vi "Eval_SglVar_MultiRes.vi"(8 "error in (no error)":errorcluster, 9 "varValue":dbl format="%#_13g", 11 "muExpr in":refnum<class "mupExpr.lvclass">) -> (0 "error out":errorcluster, 2 "Results":dbl[](array[numeric]), 3 "muExpr out":refnum<class "mupExpr.lvclass">)   [LabVIEW 2015, in "mupExpr.lvclass"]
doc: "Updates the value of the selected single variable then evaluates all expressions. Returns one result per expression.\n\nIf the expressions contain no variables, the input value is ignored.\n\nIf the expressions contain more than one variable only the \"Single Variable\" is updated.\n\nIf the variables are defined for bulk mode evaluation, only the first set (index 0) will be updated and evaluated."
uses:
  mupExpr.lvclass
  mupExpr.lvclass/mupExpr.ctl
  mupLib/mupCheckError.vi
  mupLib/mupLibPath.vi
  <vilib>/Utility/error.llb/Error Cluster From Error Code.vi
  mupLib/mupLib.lvlib
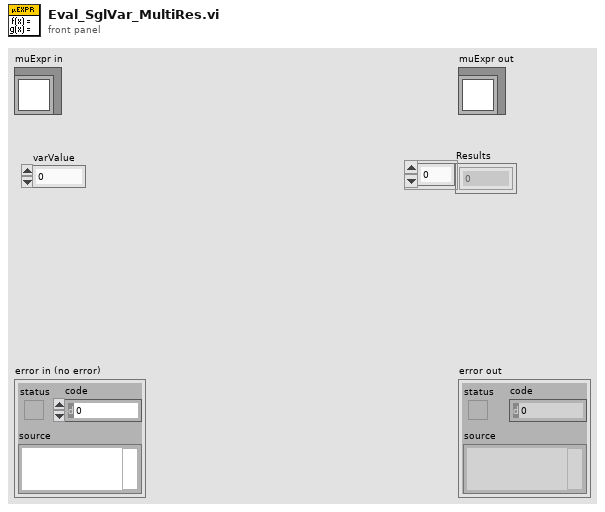
[diagram p1: front panel]
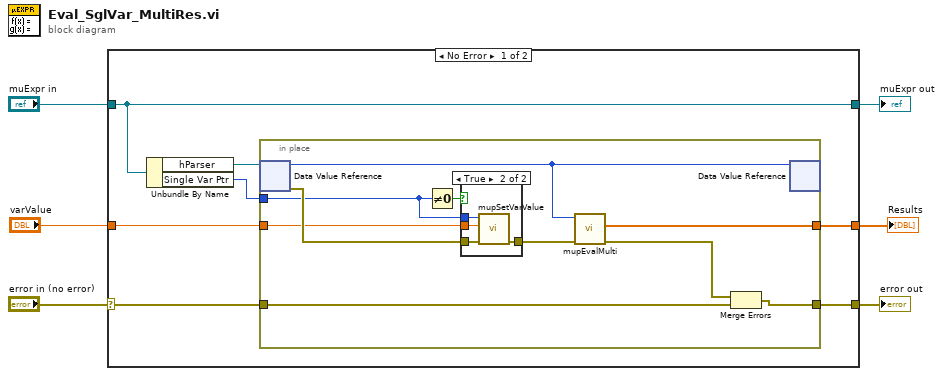
[diagram p0: block diagram]
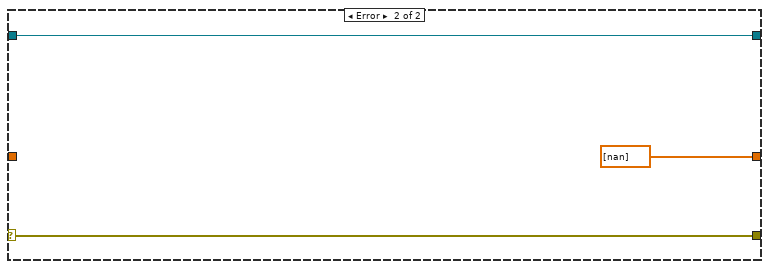
[diagram p3: hidden frame]
diagram:
  n1 = case shown="No Error" "error in (no error)" {
    selector: "error in (no error)" -> [w13 w31]
    tunnel: [w11 w31] -> w5
    tunnel: [w7 w30] -> w3
    tunnel: "muExpr in" -> [w7 w30]
    tunnel: "varValue" -> [w12 _]
    tunnel: [w10 dbl[] [nan] ("results")] -> w1
    frame No Error {
      n2 = Unbundle By Name(w7) -> ("hParser"=w9:refnum<data-value>, "Single Var Ptr"=w8:u64)
      n3 = in-place {
        in-place-border: w13 -> [w22]
        in-place-border: w12 -> [w16]
        in-place-border: [w20] -> w11
        in-place-border: [w23] -> w10
        in-place-border: w8 -> [w14]
        n4 = in-place-dvr #1(w9) -> (w15:u64, w17:errorcluster)
        n5 = Not Equal To 0?(x=w14) -> (x != 0?=w19:bool)
        n6 = case shown="True" w19 {
          tunnel: w17 -> [w24 w28]
          tunnel: w16 -> [_ w27]
          tunnel: [w24 w26] -> w18
          tunnel: w14 -> [_ w25]
          frame False {
          }
          frame True {
            n7 = call "mupSetVarValue.vi"("error in (no error)"=w28, "varValue"=w27, "varAddr in"=w25) -> ("error out"=w26:errorcluster)  [unwired: 7 in, 1 out]
          }
        }
        n8 = call "mupEvalMulti.vi"("error in (no error)"=w18, "hParser in"=w15) -> ("error out"=w21:errorcluster, "results"=w23:dbl[])  [unwired: 6 in, 2 out]
        n9 = Merge Errors(w21, w22) -> (w20:errorcluster)
        n10 = in-place-dvr #1(w15) -> ()  [unwired: 2 out]
      }
    }
    frame Error {
    }
  }
  "error out" <- w5
  "muExpr out" <- w3
  "Results" <- w1
